vi "Init.vi"(8 "error in (no error)":errorcluster, 11 "uService Template in":refnum<class "Detector Manager.lvclass">) -> (0 "error out":errorcluster, 3 "uService Template out":refnum<class "Detector Manager.lvclass">)   [LabVIEW 2026, in "TALOS.lvlib" / "Detector Manager.lvlib" / "Detector Manager.lvclass"]
uses:
  Detector Manager.lvclass
  C:/LabVIEW Code/TALOS/talos/Ancestor/Ancestor/Ancestor.lvclass
  C:/LabVIEW Code/TALOS/talos/Father of all uServices/Father of all uServices/Father of all uServices.lvclass
  Detector Manager Consumer Case Selector.ctl
  Ancestor/Ancestor/Ancestor.lvclass/Ancestor.ctl
  Father of all uServices/Father of all uServices/Father of all uServices.lvclass/Father of all uServices.ctl
  Father of all uServices/Father of all uServices Messages/Consumer Msg/Consumer Msg.lvclass/Consumer Msg.ctl
  Ancestor/Ancestor/Read ID.vi
  Support VIs/Substitute Error.vi
  Father of all uServices/Father of all uServices Messages/Consumer Msg/Send Consumer.vi
  Support VIs/Generate Error.vi
  FGV/Error Memory/Get Error Description.vi
  Support VIs/Get PC name.vi
  Support VIs/Get Class Name.vi
  <vilib>/Utility/error.llb/Clear Errors.vi
  FGV/Error Memory/Error Memory Core.vi
  <vilib>/AdvancedString/Delimited String to 1D String Array.vi
  <vilib>/AdvancedString/Delimited String to 1D String Array (string).vi
  Support VIs/Circus Root Path.vi
  FGV/Error Memory/Error Crt Lvl checker.vi
  FGV/Error Memory/Error Memory Core.vi/40c8088d-b597-4017-91af-faa98e00292e.vi
  FGV/Error Memory/Error Memory Core.vi/d4a3ab98-063c-4e44-b43d-fbdcfe6c2be2.vi
  Father of all uServices/Father of all uServices/Father of all uServices.lvclass
  C:/LabVIEW Code/TALOS/builds/Actor Framework PPL/Actor Framework.lvlibp/1abvi3w/vi.lib/ActorFramework/Actor/Actor.lvclass
  Support VIs/Global Memory.vi
  <vilib>/Utility/LVClass/Get LV Class Name.vi
  Support VIs/Is in Packed Library.vi
  Support VIs/TALOS Root path.vi
  Support VIs/Read CSV worksheet.vi
  Support VIs/Global Constants.vi
  <vilib>/Utility/error.llb/General Error Handler.vi
  Support VIs/Error Log.vi
  builds/Actor Framework PPL/Actor Framework.lvlibp/1abvi3w/vi.lib/ActorFramework/Actor/Read Self Enqueuer.vi
  <userlib>/_OpenG.lib/lvdata/lvdata.llb/Get Strings from Enum__ogtk.vi
  builds/Actor Framework PPL/Actor Framework.lvlibp/1abvi3w/vi.lib/ActorFramework/Message Enqueuer/Enqueue.vi
  Ancestor/Ancestor/Ancestor.lvclass
  <vilib>/Comparison/Equal/Equal Functor/Equal Functor.lvclass
  Father of all uServices/Father of all uServices Messages/Consumer Msg/Consumer Msg.lvclass
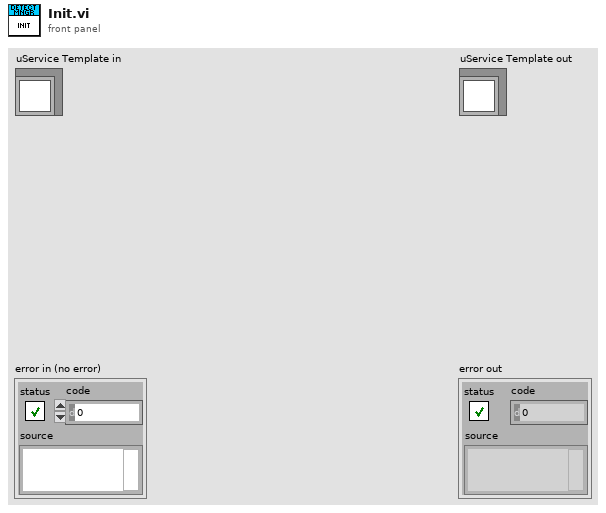
[diagram p1: front panel]
types:
  T1 = typedef "TALOS.lvlib/Detector Manager.lvlib/Detector Manager.lvclass/Detector Manager Consumer Case Selector.ctl" = enum16{"Set Configuration", "Arm", "Acquiring", "Save Data", "Self Check", "Safe Mode", "Init", "Close", "Stop"}
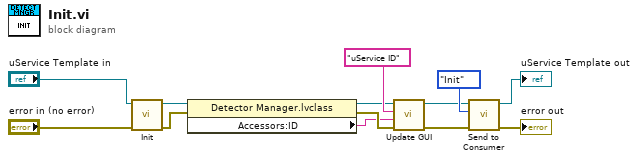
[diagram p0: block diagram]
diagram:
  n1 = call-parent "Init.vi"("error in (no error)"="error in (no error)", "uService Template in"="uService Template in") -> ("error out"=w6:errorcluster, "uService Template out"=w7:refnum<class "Detector Manager.lvclass">)  [unwired: 8 in]
  n2 = property class="Detector Manager.lvclass"(reference=w7, error in=w6) -> (reference out=w5:refnum<class "Detector Manager.lvclass">, error out=w4:errorcluster, "Accessors:ID"=w3:string)
  n3 = call "Update GUI.vi"("error in (no error)"=w4, "Data"=w3, "GUI Item Name"="uService ID", "uService Template in"=w5) -> ("error out"=w2:errorcluster, "uService Template out"=w1:refnum<class "Detector Manager.lvclass">)  [unwired: 6 in]
  n4 = call "Send to Consumer.vi"("error in (no error)"=w2, "Case ID"=Detector_Manager_Consumer_Case_Selector."Init" ("Detector Manager Consumer Case Selector"), "uService Template in"=w1) -> ("error out"=→"error out":errorcluster, "uService Template out"=→"uService Template out":refnum<class "Detector Manager.lvclass">)  [unwired: 7 in]
